vi "Query OPC.vi"(8 "error in (no error)":errorcluster, 11 "VISA resource name":refnum<visa-resource-name>) -> (0 "error out":errorcluster, 2 "OPC":i32, 3 "VISA resource name out":refnum<visa-resource-name>)   [LabVIEW 2020, in "Rohde&Schwarz CMWXP NR FR1 Measurement.lvlib"]
doc: "This VI sends OPC query to the instrument. This effectively causes your program to wait in this VI until the instrument has processed all the commands you have sent to it until this point. Use the VI to force the synchronization of the instrument with you program.\n\nAttribute:\n-\n\nRemote-control command:\n*OPC?"
uses:
  <instrlib>/Rohde&Schwarz CMWXP NR FR1 Measurement/Rohde&Schwarz CMWXP NR FR1 Measurement.lvlib
  <instrlib>/Rohde&Schwarz CMWXP NR FR1 Measurement/Private/rsidr_core.llb/rsidr_core.lvlib
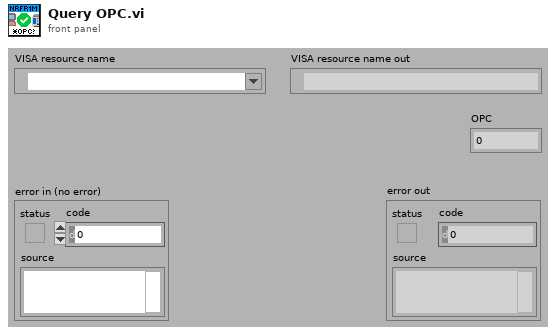
[diagram p1: front panel]
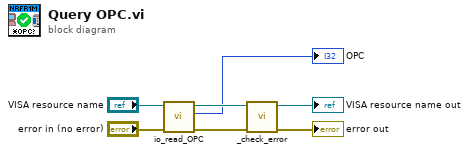
[diagram p0: block diagram]
diagram:
  n1 = call <instrlib>:"io_read_OPC.vi"("error in"="error in (no error)", "VISA resource name"="VISA resource name") -> ("error out"=w7:errorcluster, "OPC returned"=→"OPC":i32, "VISA resource name out"=w6:refnum<visa-resource-name>)  [unwired: 7 in]
  n2 = call <instrlib>:"_check_error.vi"("error in (no error)"=w7, "VISA resource name"=w6) -> ("error out"=→"error out":errorcluster, "VISA resource name out"=→"VISA resource name out":refnum<visa-resource-name>)  [unwired: 8 in]
